vi "ASM.Event.Start.vi"(8 "error in (no error)":errorcluster, 11 "ActorStateMachine in":refnum<class "ActorStateMachine.lvclass">) -> (0 "error out":errorcluster, 3 "ActorStateMachine out":refnum<class "ActorStateMachine.lvclass">)   [LabVIEW 2021, in "ActorStateMachine.lvlib" / "ActorStateMachine.lvclass"]
uses:
  ActorStateMachine.lvclass
  ActorStateMachine.lvclass/ActorStateMachine.ctl
  _ASM.State.ctl
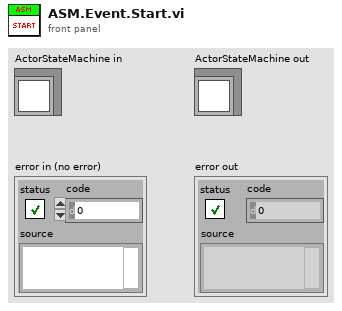
[diagram p1: front panel]
types:
  T1 = typedef "ActorStateMachine.lvlib/ActorStateMachine.lvclass/_ASM.State.ctl" = enum16{"Boom", "Pre-Init", "Init", "Post-Init", "Pre-Reset", "Reset", "Post-Reset", "Pre-Config", "Config", "Post-Config", "Pre-Ready", "Ready", "Post-Ready", "Pre-Running", "Running", "Next", "Post-Running", "Break", "Fail", "Crash", "Shutdown", "Doom"}
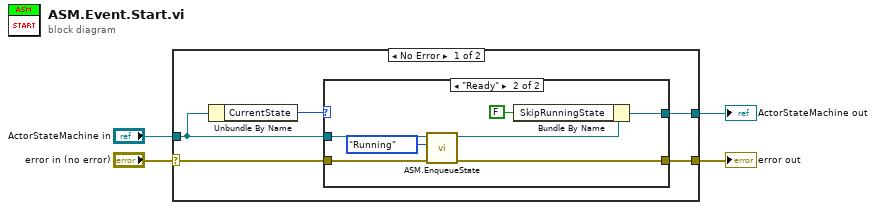
[diagram p0: block diagram]
diagram:
  n1 = case shown="No Error" "error in (no error)" {
    selector: "error in (no error)" -> [w8 w20]
    tunnel: [w9 w20] -> w2
    tunnel: [w6 w19] -> w1
    tunnel: "ActorStateMachine in" -> [w5 w19]
    frame No Error {
      n2 = Unbundle By Name(w5) -> ("CurrentState"=w7:T1)
      n3 = case shown="\"Ready\"" w7 {
        tunnel: [w11 w17] -> w9
        tunnel: w8 -> [w11 w18]
        tunnel: w5 -> [w10 w16]
        tunnel: [w10 w13] -> w6
        frame Default {
        }
        frame "Ready" {
          n4 = call "ASM.EnqueueState.vi"("error in (no error)"=w18, "NextState"=_ASM.State."Running", "ActorStateMachine in"=w16) -> ("error out"=w17:errorcluster, "ActorStateMachine out"=w14:refnum<class "ActorStateMachine.lvclass">)  [unwired: 7 in]
          n5 = Bundle By Name(cluster=w14, "SkipRunningState"=FALSE) -> (w13:refnum<class "ActorStateMachine.lvclass">)
        }
      }
    }
    frame Error {
    }
  }
  "error out" <- w2
  "ActorStateMachine out" <- w1
